vi "BlockShot.vi"(0 "object in":refnum<class "DefendAreaTactic.lvclass">, 2 "Robot":refnum<class "Robot.lvclass">, 4 "Game":refnum<class "Game.lvclass">, 5 "error in (no error)":errorcluster, 7 "first call?":bool) -> (14 "object out":refnum<class "DefendAreaTactic.lvclass">, 16 "Robot out":refnum<class "Robot.lvclass">, 19 "error out":errorcluster)   [LabVIEW 2024, in "DefendAreaTactic.lvclass"]
uses:
  DefendAreaTactic.lvclass
  Robot_class/Robot.lvclass
  C:/Users/ROBOIME2/Documents/SSL ROBOIME/SSL_AI/Object_class/Object.lvclass
  Game_class/Game.lvclass
  Game_class/Game.lvclass/Game.ctl
  Object_class/Object.lvclass/Object.ctl
  Parameters_class/Parameters.lvclass/Parameters.ctl
  Ball_class/Ball.lvclass/Ball.ctl
  Field_class/Field.lvclass/Field.ctl
  Robot_class/Robot.lvclass/Robot.ctl
  Field_class/Read ourGoalPosition.vi
  Parameters_class/Read KickForce.vi
  Parameters_class/Read ChipKick Force 1.vi
  Object_class/Read position(x,y).vi
  Ball_class/Read v_x.vi
  Ball_class/Read v_y.vi
  Ball_class/Read velocityNorm.vi
  Robot_class/Write dest_vel.vi
  Robot_class/Write dest_x.vi
  Robot_class/Write dest_y.vi
  Robot_class/Write dest_orientation.vi
  Robot_class/Write kick_x.vi
  Robot_class/Write kick_z.vi
  Game_class/Read FieldRef.vi
  Game_class/Read BallRef.vi
  Game_class/Read Parameters.lvclass.vi
  <vilib>/Analysis/_algsub.llb/Vector Norm.vi
  <vilib>/Analysis/_algsub.llb/Real Vector Norm.vi
  Ball_class/Ball.lvclass
  Field_class/Field.lvclass
  Parameters_class/Parameters.lvclass
  Utilities_class/Utilities.lvclass
  <vilib>/Analysis/NI_AALPro.lvlib
  DefendGoalTactic_class/DefendGoalTactic.lvclass
  <vilib>/Analysis/NI_AALBLAS.lvlib
  <vilib>/Analysis/coordinate.llb/2D Cartesian Coordinate Rotation (Scalar).vi
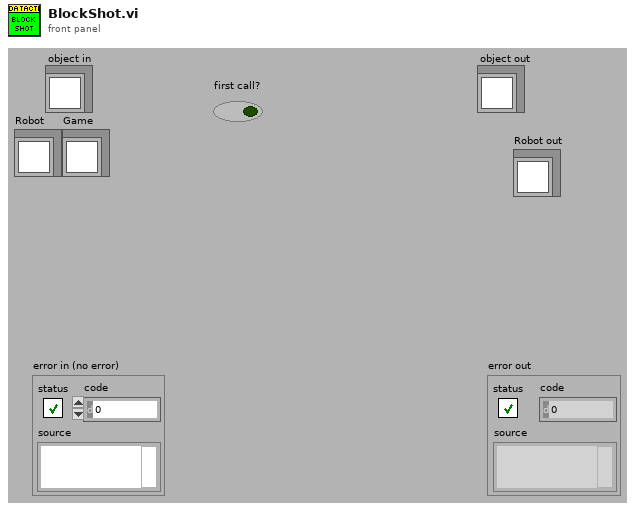
[diagram p1: front panel]
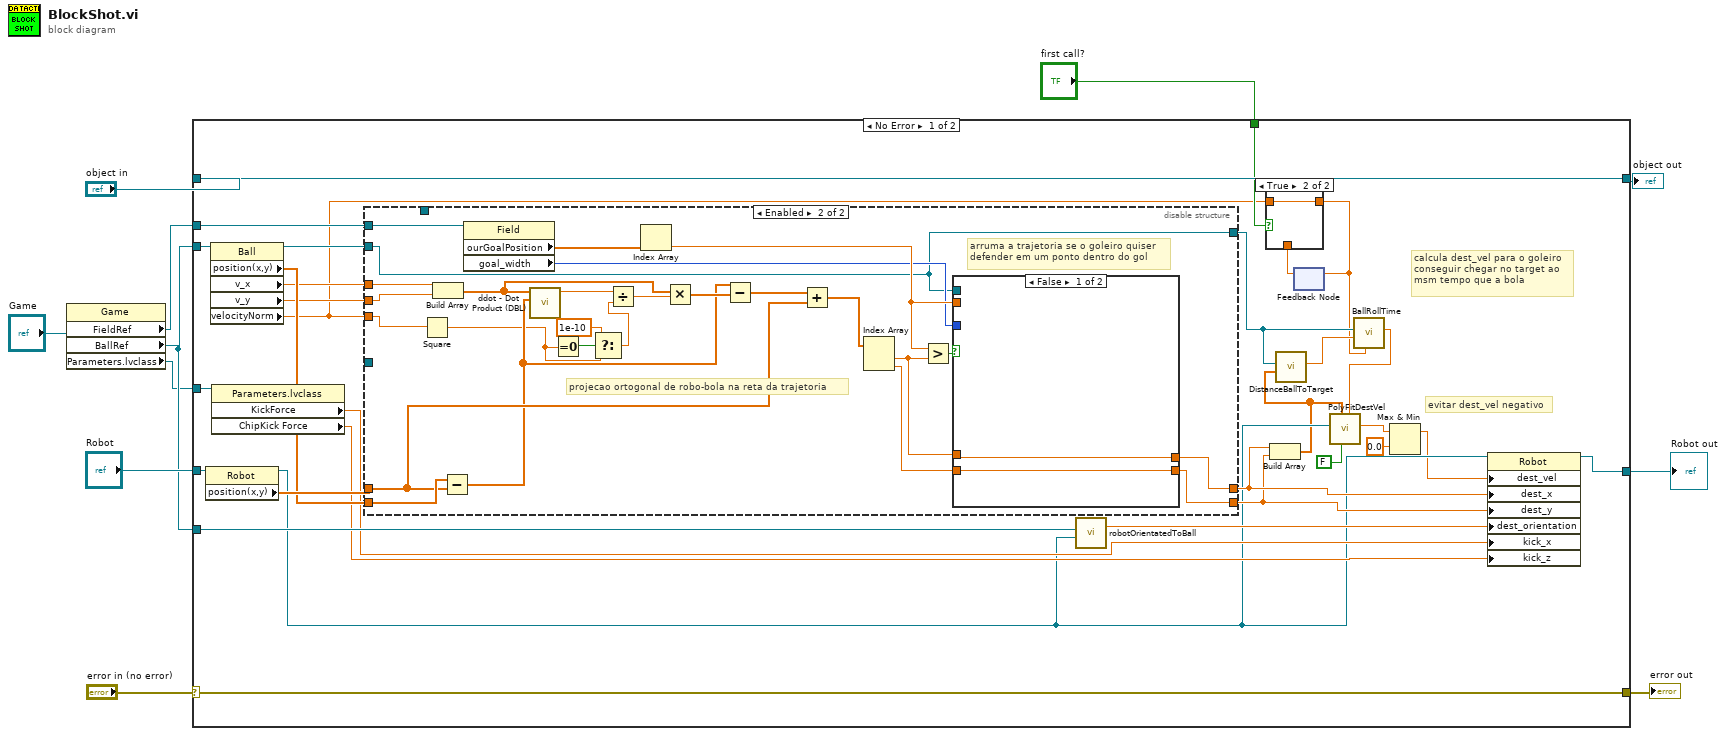
[diagram p0: block diagram]
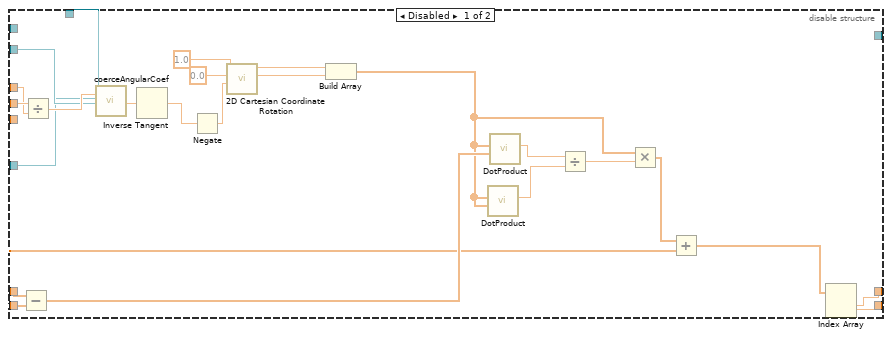
[diagram p3: hidden frame]
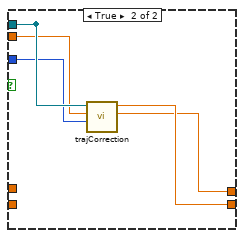
[diagram p4: hidden frame]
diagram:
  n1 = property class="Game"(reference="Game") -> ("FieldRef"=w3:refnum<class "Field.lvclass">, "BallRef"=w4:refnum<class "Ball.lvclass">, "Parameters.lvclass"=w2:refnum<class "Parameters.lvclass">)  [unwired: 1 in, 2 out]
  n2 = case shown="No Error" "error in (no error)" {
    selector: "error in (no error)" -> [w42 w104]
    tunnel: [w42 w104] -> w10
    tunnel: [w37 w103] -> w8
    tunnel: "object in" -> [w37 w103]
    tunnel: "Robot" -> [w41 w102]
    tunnel: w4 -> [w40 _]
    tunnel: [w39 w102] -> w5
    tunnel: w4 -> [w34 _]
    tunnel: w3 -> [w33 _]
    tunnel: w2 -> [w31 _]
    tunnel: "first call?" -> [w18 _]
    frame No Error {
      # "calcula dest_vel para o goleiro\nconseguir chegar no target ao\nmsm tempo que a bola"
      # "evitar dest_vel negativo"
      n3 = property class="Robot"(reference=w41) -> (reference out=w23:refnum<class "Robot.lvclass">, "position(x,y)"=w36:dbl[])  [unwired: 1 in, 1 out]
      n4 = property class="Ball"(reference=w40) -> (reference out=w32:refnum<class "Ball.lvclass">, "position(x,y)"=w35:dbl[], "v_x"=w27:dbl, "v_y"=w28:dbl, "velocityNorm"=w17:dbl)  [unwired: 1 in, 1 out]
      n5 = property class="Parameters.lvclass"(reference=w31) -> ("KickForce"=w30:dbl, "ChipKick Force"=w29:dbl)  [unwired: 1 in, 2 out]
      n6 = disable-structure shown="Enabled" {
        disable-tunnel: _ -> [w67 _]
        disable-tunnel: w32 -> [w66 w69]
        disable-tunnel: _ -> [w65 _]
        disable-tunnel: w28 -> [w59 w93]
        disable-tunnel: w27 -> [w58 w94]
        disable-tunnel: w36 -> [w57 w84]
        disable-tunnel: w35 -> [w51 w85]
        disable-tunnel: [w48 w76] -> w25
        disable-tunnel: [w47 w75] -> w24
        disable-tunnel: w17 -> [_ w92]
        disable-tunnel: w33 -> [_ w79]
        disable-tunnel: [_ w69] -> w22
        frame Disabled {
          n7 = Subtract(x=w57, y=w51) -> (x-y=w56:dbl[])
          n8 = Divide(x=w59, y=w58) -> (x/y=w68:dbl)
          n9 = call "coerceAngularCoef.vi"("object in"=w67, "Coef ang"=w68, "Field"=w65, "Ball"=w66) -> ("coerced(x)"=w62:dbl)  [unwired: 13 in, 2 out]
          n10 = Inverse Tangent(1:w62) -> (0:w46:dbl)
          n11 = Negate(x=w46) -> (-x=w45:dbl)
          n12 = call-poly <vilib>:"2D Cartesian Coordinate Rotation.vi"("theta"=w45, "y"=0.0, "x"=1.0) -> ("y out"=w60:dbl, "x out"=w61:dbl)  [unwired: 6 in, 1 out]
          n13 = Build Array(w61, w60) -> (w52:dbl[])
          n14 = call "DotProduct.vi"("Point2"=w52, "Point1"=w52) -> ("dot product"=w54:dbl)  [unwired: 7 in, 2 out]
          n15 = call "DotProduct.vi"("Point2"=w56, "Point1"=w52) -> ("dot product"=w55:dbl)  [unwired: 7 in, 2 out]
          n16 = Divide(x=w55, y=w54) -> (x/y=w53:dbl)
          n17 = Multiply(x=w52, y=w53) -> (x*y=w50:dbl[])
          n18 = Add(x=w50, y=w51) -> (x+y=w49:dbl[])
          n19 = Index Array(array=w49) -> (element #1=w48:dbl, element #2=w47:dbl)  [unwired: 2 in]
        }
        frame Enabled {
          # "arruma a trajetoria se o goleiro quiser \ndefender em um ponto dentro do gol"
          # "projecao ortogonal de robo-bola na reta da trajetoria"
          n20 = Square(x=w92) -> (x^2=w72:dbl)
          n21 = Build Array(w94, w93) -> (w89:dbl[])
          n22 = Subtract(x=w85, y=w84) -> (x-y=w83:dbl[])
          n23 = property class="Field"(reference=w79) -> ("ourGoalPosition"=w78:dbl[], "goal_width"=w74:i32)  [unwired: 1 in, 2 out]
          n24 = call <vilib>:"ddot - Dot Product (DBL).vi"("y"=w83, "x"=w89) -> ("ddot"=w91:dbl)  [unwired: 8 in, 1 out]
          n25 = Equal To 0?(x=w72) -> (x = 0?=w73:bool)
          n26 = Select(t=1e-10, s=w73, f=w72) -> (s? t:f=w71:dbl)
          n27 = Divide(x=w91, y=w71) -> (x/y=w90:dbl)
          n28 = Index Array(array=w78) -> (element=w77:dbl)  [unwired: 1 in]
          n29 = Multiply(x=w89, y=w90) -> (x*y=w88:dbl[])
          n30 = Subtract(x=w83, y=w88) -> (x-y=w87:dbl[])
          n31 = Add(x=w87, y=w84) -> (x+y=w86:dbl[])
          n32 = Index Array(array=w86) -> (element #1=w80:dbl, element #2=w81:dbl)  [unwired: 2 in]
          n33 = Greater?(x=w77, y=w80) -> (0:w82:bool)
          n34 = case shown="False" w82 {
            tunnel: w81 -> [w95 _]
            tunnel: w80 -> [w96 _]
            tunnel: w77 -> [_ w100]
            tunnel: [_ w101] -> _
            tunnel: w69 -> [_ w101]
            tunnel: [w96 w98] -> w76
            tunnel: [w95 w99] -> w75
            tunnel: w74 -> [_ w97]
            frame False {
            }
            frame True {
              n35 = call "trajCorrection.vi"("goal Width"=w97, "goal X"=w100, "BallRef"=w101) -> ("x"=w98:dbl, "y"=w99:dbl)  [unwired: 6 in]
            }
          }
        }
      }
      n36 = call "robotOrientatedToBall.vi"("Robot"=w23, "BallRef"=w34) -> ("Orientation"=w38:dbl)  [unwired: 7 in, 2 out]
      n37 = Build Array(w25, w24) -> (w21:dbl[])
      n38 = call "DistanceBallToTarget.vi"("Target"=w21, "Ball"=w22) -> ("Distance Ball To Target"=w20:dbl)  [unwired: 7 in, 2 out]
      n39 = feedback #1() -> (w16:dbl)  [unwired: 1 in]
      n40 = case shown="True" w18 {
        tunnel: w17 -> [_ w44]
        tunnel: [w43 w44] -> w15
        tunnel: w16 -> [w43 _]
        frame False {
        }
        frame True {
        }
      }
      n41 = feedback-in #1(w15) -> ()
      n42 = call "BallRollTime.vi"("v_ini"=w15, "distance"=w20, "Ball"=w22) -> ("time"=w19:dbl)  [unwired: 6 in, 2 out]
      n43 = call "PolyFitDestVel.vi"("TargetTime"=w19, "use model?"=FALSE, "TargetPos"=w21, "Robot"=w23) -> ("vf"=w13:dbl)  [unwired: 5 in, 2 out]
      n44 = Max & Min(x=w13, y=0.0) -> (max(x,y)=w12:dbl)  [unwired: 1 out]
      n45 = property class="Robot"(reference=w23, "dest_vel"=w12, "dest_x"=w25, "dest_y"=w24, "dest_orientation"=w38, "kick_x"=w30, "kick_z"=w29) -> (reference out=w39:refnum<class "Robot.lvclass">)  [unwired: 1 in, 1 out]
    }
    frame Error {
    }
  }
  "error out" <- w10
  "object out" <- w8
  "Robot out" <- w5
